vi "fgv_pc_rplidar.vi"(7 "cmd":T1, 8 "error in":errorcluster) -> (0 "error out":errorcluster, 2 "serial buf":u32, 3 "read buffer":string)   [LabVIEW 2019]
uses:
  Ctrl/rplidar_cmd.ctl
  <vilib>/Instr/_visa.llb/VISA Configure Serial Port (Instr).vi
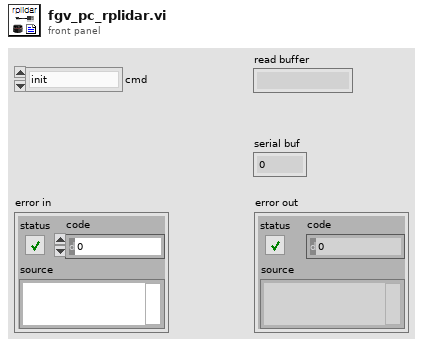
[diagram p1: front panel]
types:
  T1 = typedef "rplidar_cmd.ctl" = enum16{"init", "health", "spin", "scan", "read", "stop", "close"}
  T2 = typedef "system_hw.ctl" = cluster{"AGV":enum16{"none", "ERP42", "ERP42mini", "Scout", "Ycar"}, "Lidar 1":enum16{"none", "VLP16", "TIM571", "RPLidar A2", "RPLidar A3"}, "Lidar 2":enum16{"none", "VLP16", "TIM571", "RPLidar A2", "RPLidar A3"}, "GPS":enum16{"none", "F9P", "M8P", "PwrPak7", "19X HVS"}, "Camera":enum16{"none", "C920", "C922", "GT1290C", "MS LifeCam"}, "Joystick":enum16{"none", "joystick"}, "sound":enum16{"none", "speaker"}, "IMU":enum16{"none", "MW-AHRSv1"}}
  T3 = enum16{"none", "VLP16", "TIM571", "RPLidar A2", "RPLidar A3"}
  T4 = cluster{"port":refnum<visa-resource-name>, "dt":u32, "update n":u8, "speed":u16, "rate ":u32}
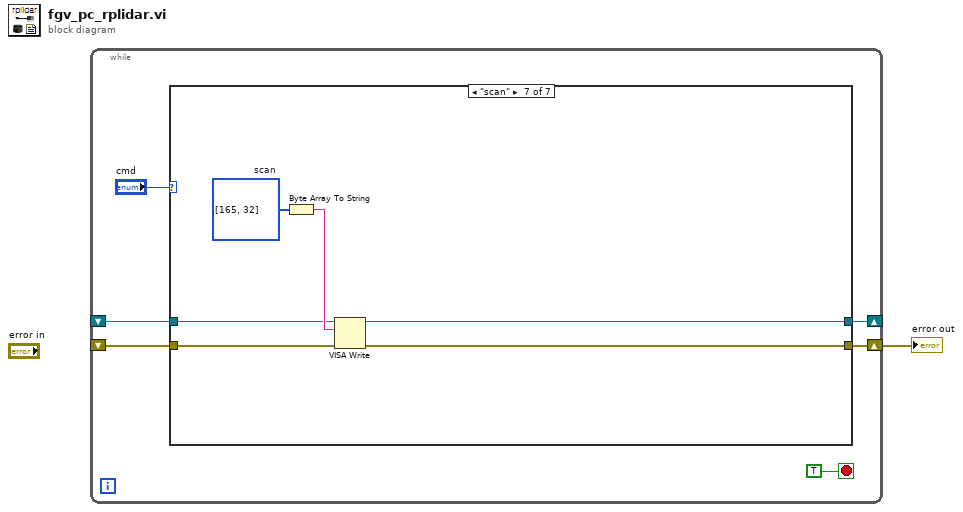
[diagram p0: block diagram]
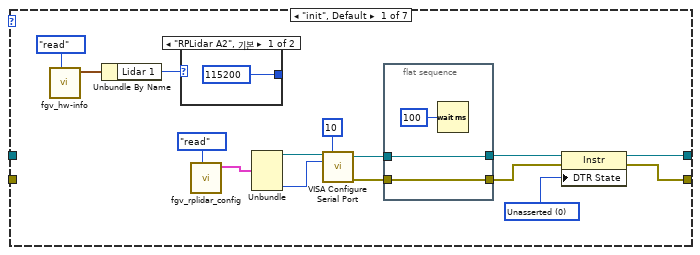
[diagram p2: hidden frame]
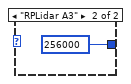
[diagram p3: hidden frame]
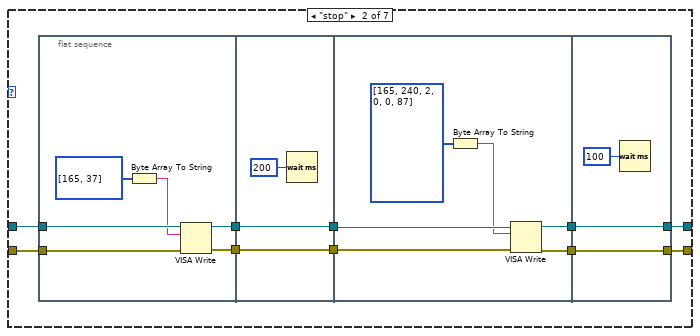
[diagram p4: hidden frame]
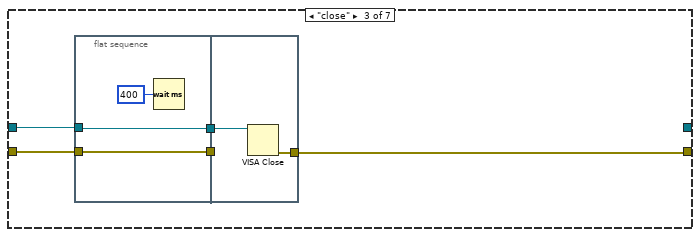
[diagram p5: hidden frame]
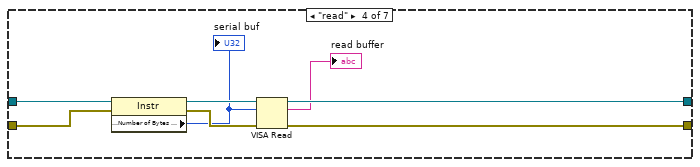
[diagram p6: hidden frame]
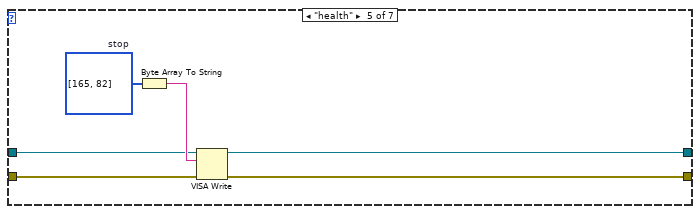
[diagram p7: hidden frame]
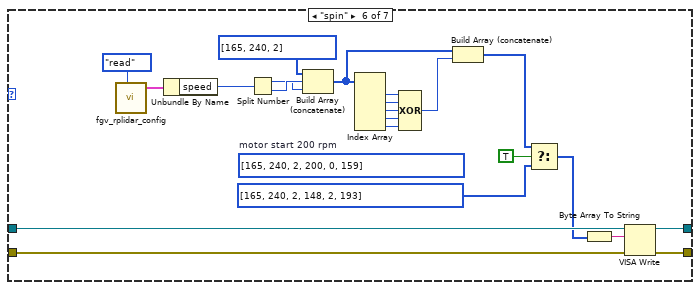
[diagram p8: hidden frame]
diagram:
  n1 = while {
    shift-right: [w4] -> _
    shift-left: _ -> [w2]
    shift-right: [w5] -> w1
    shift-left: _ -> [w3]
    stop <- TRUE stop-if-true
    n2 = case shown="\"scan\"" "cmd" {
      tunnel: [w16 w29 w58 w69 w75 w98 w102] -> w5
      tunnel: [w15 w28 _ w68 w74 w97 w103] -> w4
      tunnel: w3 -> [_ w30 w59 w73 w76 w99 w104]
      tunnel: w2 -> [_ w31 w60 w72 w77 w100 w105]
      frame "init", Default {
        w18 = i16 0 items=["Unknown"=-1, "Unasserted"=0, "Asserted"=1] ("Serial Settings:Modem Line Settings:Line DTR State")
        n3 = call "fgv_hw-info.vi"("cmd"=enum16{"write", "read"}."read") -> ("HW info out"=w10:T2)  [unwired: 10 in]
        n4 = Unbundle By Name(w10) -> ("Lidar 1"=w9:T3)
        n5 = case shown="\"RPLidar A2\", 기본" w9 {
          tunnel: [u32 115200 ("baud rate (9600)") u32 256000 ("baud rate (9600)")] -> _
          frame "RPLidar A2", Default {
          }
          frame "RPLidar A3" {
          }
        }
        n6 = call "fgv_rplidar_config.vi"("cmd"=enum16{"read", "write"}."read") -> ("RPLidar cfg out"=w13:T4)  [unwired: 9 in, 1 out]
        n7 = Unbundle(w13) -> ("port"=w12:refnum<visa-resource-name>, "rate"=w8:u32)  [unwired: 3 out]
        n8 = call-poly "VISA Configure Serial Port"("VISA resource name"=w12, "timeout (10sec)"=u32 10, "baud rate (9600)"=w8) -> ("VISA resource name out"=w22:refnum<visa-resource-name>, "error out"=w21:errorcluster)  [unwired: 11 in]
        n9 = flat-sequence {
          tunnel: [w26] -> w20
          tunnel: w22 -> [w26]
          tunnel: [w25] -> w19
          tunnel: w21 -> [w25]
          frame #0 {
            n10 = Wait (ms)(milliseconds to wait=u32 100) -> ()  [unwired: 1 out]
          }
        }
        n11 = property class="Instr"(reference=w20, error in=w19, "DTR State"=w18) -> (reference out=w15:refnum<visa-resource-name>, error out=w16:errorcluster)
      }
      frame "stop" {
        n12 = flat-sequence {
          tunnel: [w41] -> w37
          tunnel: [w40] -> w36
          tunnel: w31 -> [w43]
          tunnel: w30 -> [w42]
          tunnel: w37 -> [w46]
          tunnel: [w46] -> w35
          tunnel: w36 -> [w45]
          tunnel: [w45] -> w34
          tunnel: w35 -> [w52]
          tunnel: w34 -> [w51]
          tunnel: [w50] -> w33
          tunnel: [w49] -> w32
          tunnel: w33 -> [w55]
          tunnel: w32 -> [w54]
          tunnel: [w55] -> w28
          tunnel: [w54] -> w29
          frame #0 {
            n13 = Byte Array To String(unsigned byte array=u8[] [165, 37] ("appended array")) -> (string=w38:string)
            n14 = VISA Write(VISA resource name=w43, write buffer=w38, error in (no error)=w42) -> (VISA resource name out=w41:refnum<visa-resource-name>, error out=w40:errorcluster)  [unwired: 1 out]
          }
          frame #1 {
            n15 = Wait (ms)(milliseconds to wait=u32 200) -> ()  [unwired: 1 out]
          }
          frame #2 {
            n16 = Byte Array To String(unsigned byte array=u8[] [165, 240, 2, 0, 0, 87] ("appended array 2")) -> (string=w47:string)
            n17 = VISA Write(VISA resource name=w52, write buffer=w47, error in (no error)=w51) -> (VISA resource name out=w50:refnum<visa-resource-name>, error out=w49:errorcluster)  [unwired: 1 out]
          }
          frame #3 {
            n18 = Wait (ms)(milliseconds to wait=u32 100) -> ()  [unwired: 1 out]
          }
        }
      }
      frame "close" {
        n19 = flat-sequence {
          tunnel: [w63] -> w57
          tunnel: [w62] -> w56
          tunnel: w60 -> [w63]
          tunnel: w59 -> [w62]
          tunnel: w57 -> [w65]
          tunnel: w56 -> [_]
          tunnel: [w64] -> w58
          frame #0 {
            n20 = Wait (ms)(milliseconds to wait=u32 400) -> ()  [unwired: 1 out]
          }
          frame #1 {
            n21 = VISA Close(VISA resource name=w65) -> (error out=w64:errorcluster)  [unwired: 1 in]
          }
        }
      }
      frame "read" {
        n22 = property class="Instr"(reference=w72, error in=w73) -> (reference out=w70:refnum<visa-resource-name>, error out=w71:errorcluster, "Serial Settings:Number of Bytes at Serial Port"=w67:u32)
        "serial buf" <- w67
        n23 = VISA Read(VISA resource name=w70, byte count=w67, error in (no error)=w71) -> (VISA resource name out=w68:refnum<visa-resource-name>, read buffer=→"read buffer":string, error out=w69:errorcluster)  [unwired: 1 out]
      }
      frame "health" {
        w79 = u8[] [165, 82]  # stop
        n24 = Byte Array To String(unsigned byte array=w79) -> (string=w78:string)
        n25 = VISA Write(VISA resource name=w77, write buffer=w78, error in (no error)=w76) -> (VISA resource name out=w74:refnum<visa-resource-name>, error out=w75:errorcluster)  [unwired: 1 out]
      }
      frame "spin" {
        (unwired) u8[] [165, 240, 2, 200, 0, 159]  # motor start 200 rpm
        n26 = call "fgv_rplidar_config.vi"("cmd"=enum16{"read", "write"}."read") -> ("RPLidar cfg out"=w81:T4)  [unwired: 9 in, 1 out]
        n27 = Unbundle By Name(w81) -> ("speed"=w80:u16)
        n28 = Split Number(x=w80) -> (hi(x)=w84:u8, lo(x)=w85:u8)
        n29 = Build Array (concatenate)(u8[] [165, 240, 2] ("packet 3"), w85, w84) -> (w87:u8[])
        n30 = Index Array(array=w87) -> (element #1=w93:u8, element #2=w92:u8, element #3=w91:u8, element #4=w90:u8, element #5=w88:u8)  [unwired: 5 in]
        n31 = Compound Arithmetic op=XOR(w93, w92, w91, w90, w88) -> (w86:u8)
        n32 = Build Array (concatenate)(w87, w86) -> (w83:u8[])
        n33 = Select(t=w83, s=TRUE, f=u8[] [165, 240, 2, 148, 2, 193] ("appended array")) -> (s? t:f=w95:u8[])
        n34 = Byte Array To String(unsigned byte array=w95) -> (string=w101:string)
        n35 = VISA Write(VISA resource name=w100, write buffer=w101, error in (no error)=w99) -> (VISA resource name out=w97:refnum<visa-resource-name>, error out=w98:errorcluster)  [unwired: 1 out]
      }
      frame "scan" {
        w107 = u8[] [165, 32]  # scan
        n36 = Byte Array To String(unsigned byte array=w107) -> (string=w106:string)
        n37 = VISA Write(VISA resource name=w105, write buffer=w106, error in (no error)=w104) -> (VISA resource name out=w103:refnum<visa-resource-name>, error out=w102:errorcluster)  [unwired: 1 out]
      }
    }
  }
  "error out" <- w1
